vi "Read_XY_vectors.vi"(8 "error in (no error)":errorcluster, 11 "HIS in":refnum<class "HIS.lvclass">) -> (0 "error out":errorcluster, 1 "timedelays":dbl[](array[numeric]), 2 "wavelengths":dbl[](array[numeric]), 3 "HIS out":refnum<class "HIS.lvclass">)   [LabVIEW 2018, in "HIS.lvclass"]
uses:
  HIS.lvclass
  C:/Users/Sergey Denisov/Documents/REPS/TRANCON/Classes/DATA/DATA.lvclass
  DATA.lvclass/DATA.ctl
  HIS.lvclass/HIS.ctl
  DATA.lvclass
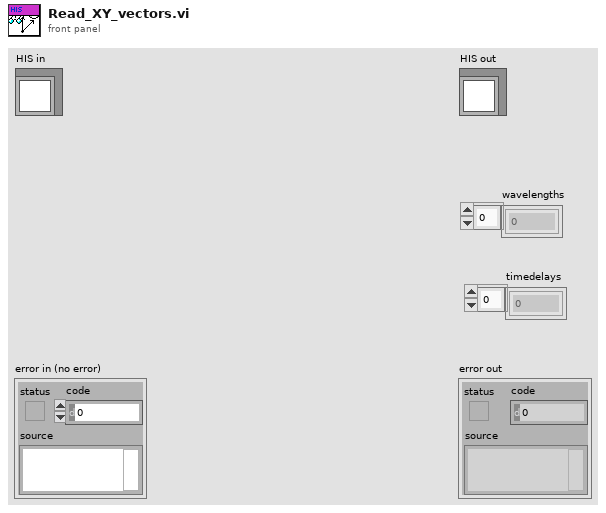
[diagram p1: front panel]
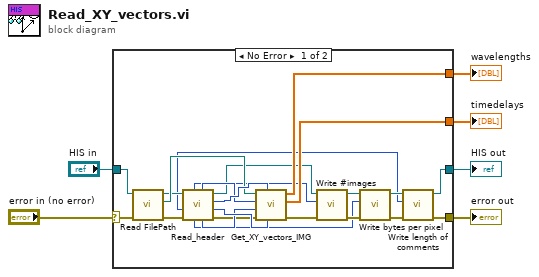
[diagram p0: block diagram]
diagram:
  n1 = case shown="No Error" "error in (no error)" {
    selector: "error in (no error)" -> [w20 w31]
    tunnel: [w7 w31] -> w5
    tunnel: [w8 w30] -> w4
    tunnel: "HIS in" -> [w24 w30]
    tunnel: [w19 _] -> w2
    tunnel: [w18 _] -> w1
    frame No Error {
      n2 = call "Read FilePath.vi"("error in (no error)"=w20, "DATA in"=w24) -> ("error out"=w22:errorcluster, "FilePath"=w23:path, "DATA out"=w21:refnum<class "HIS.lvclass">)  [unwired: 7 in]
      n3 = call "Read_header.vi"("error in (no error)"=w22, "HIS in"=w21) -> ("error out"=w25:errorcluster, "TimeDelays,pixels"=w28:i32, "Wavelength, pixels"=w29:i32, "HIS out"=w17:refnum<class "HIS.lvclass">, "ScalingYScalingFile"=w26:i64, "ScalingXScalingFile"=w27:i64, "size bytes per number"=w12:i8, "#Images"=w15:i32, "comments"=w11:u16)  [unwired: 1 in]
      n4 = call "Get_XY_vectors_IMG.vi"("TimeDelays,pixels"=w28, "Wavelength, pixels"=w29, "error in"=w25, "ScalingYScalingFile"=w26, "ScalingXScalingFile"=w27, "path"=w23) -> ("error out"=w16:errorcluster, "Y"=w18:dbl[], "X"=w19:dbl[])  [unwired: 3 in]
      n5 = call "Write #images.vi"("error in (no error)"=w16, "#images"=w15, "HIS in"=w17) -> ("error out"=w13:errorcluster, "HIS out"=w9:refnum<class "HIS.lvclass">)  [unwired: 7 in]
      n6 = call "Write bytes per pixel.vi"("error in (no error)"=w13, "bytes per pixel"=w12, "DATA in"=w9) -> ("error out"=w10:errorcluster, "DATA out"=w14:refnum<class "HIS.lvclass">)  [unwired: 7 in]
      n7 = call "Write length of comments.vi"("error in (no error)"=w10, "length of comments"=w11, "DATA in"=w14) -> ("error out"=w7:errorcluster, "DATA out"=w8:refnum<class "HIS.lvclass">)  [unwired: 7 in]
    }
    frame Error {
    }
  }
  "error out" <- w5
  "HIS out" <- w4
  "timedelays" <- w1
  "wavelengths" <- w2
